vi "Consolidate Whitespace Text Lines.vi"(1 "Input":string) -> (0 "Output (consolidated whitespace lines)":string)   [LabVIEW 2023, in "Error Manager.lvlib"]
doc: "This VI replaces any set of two or more consecutive whitespace text lines with a single whitespace text line.\n\nIn this VI whitespace is defined as: spaces, tabs, carriage returns, and linefeeds.\n\n<B>Example 1</B>\nInput:\n\"\nHello World\n\n\nHello World\n\"\n\nOutput:\n\"\nHello World\n\nHello World\n\"\n\n<B>Example 2</B>\nInput:\n\"\nHello World\n\n\nHello World\n\n\n\n\nHello World\n\"\n\nOutput:\n\"\nHello World\n\nHello World\n\nHello World\n\""
uses:
  Error Manager.lvlib
  <vilib>/Utility/error.llb/whitespace.ctl
  <vilib>/Utility/error.llb/Trim Whitespace One-Sided.vi
  OpenG VIs/OpenG VIs.lvclass
panel:
  out "Whitespace Line Indexes":i32[](array[numeric])
  # "Development\nControls or indicators that are useful for development or testing, but which are not outputs of the VI."
  # "Input\nInputs to the VI"
  # "Output\nOutputs of the VI"
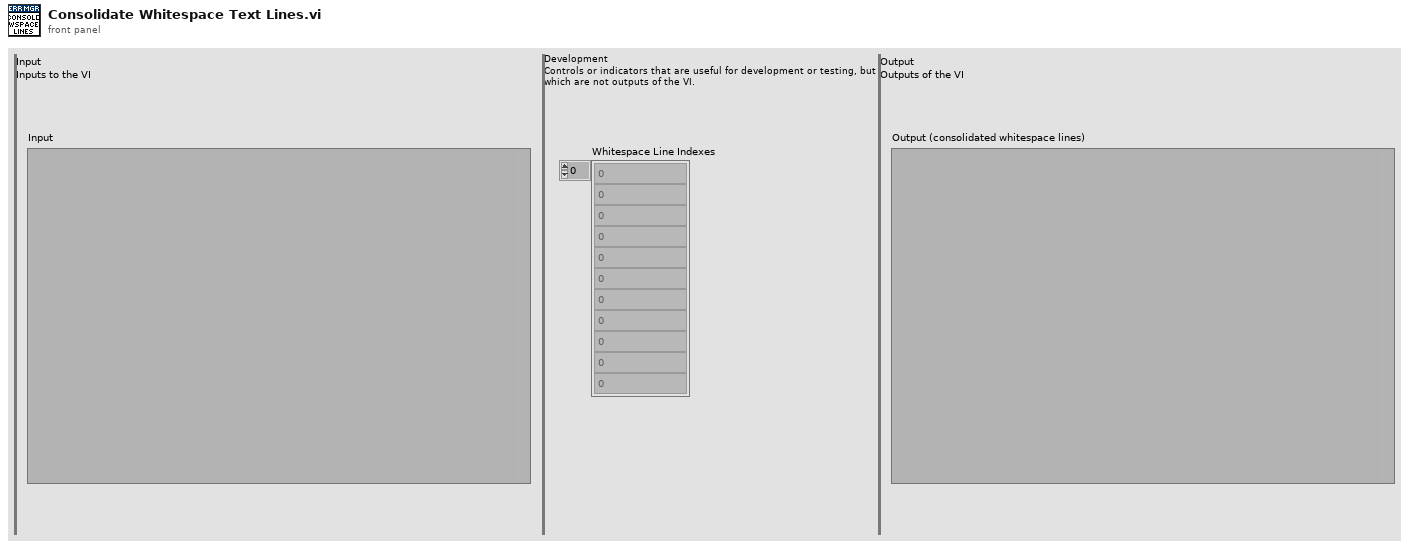
[diagram p1: front panel]
types:
  T1 = typedef "whitespace.ctl" = u16
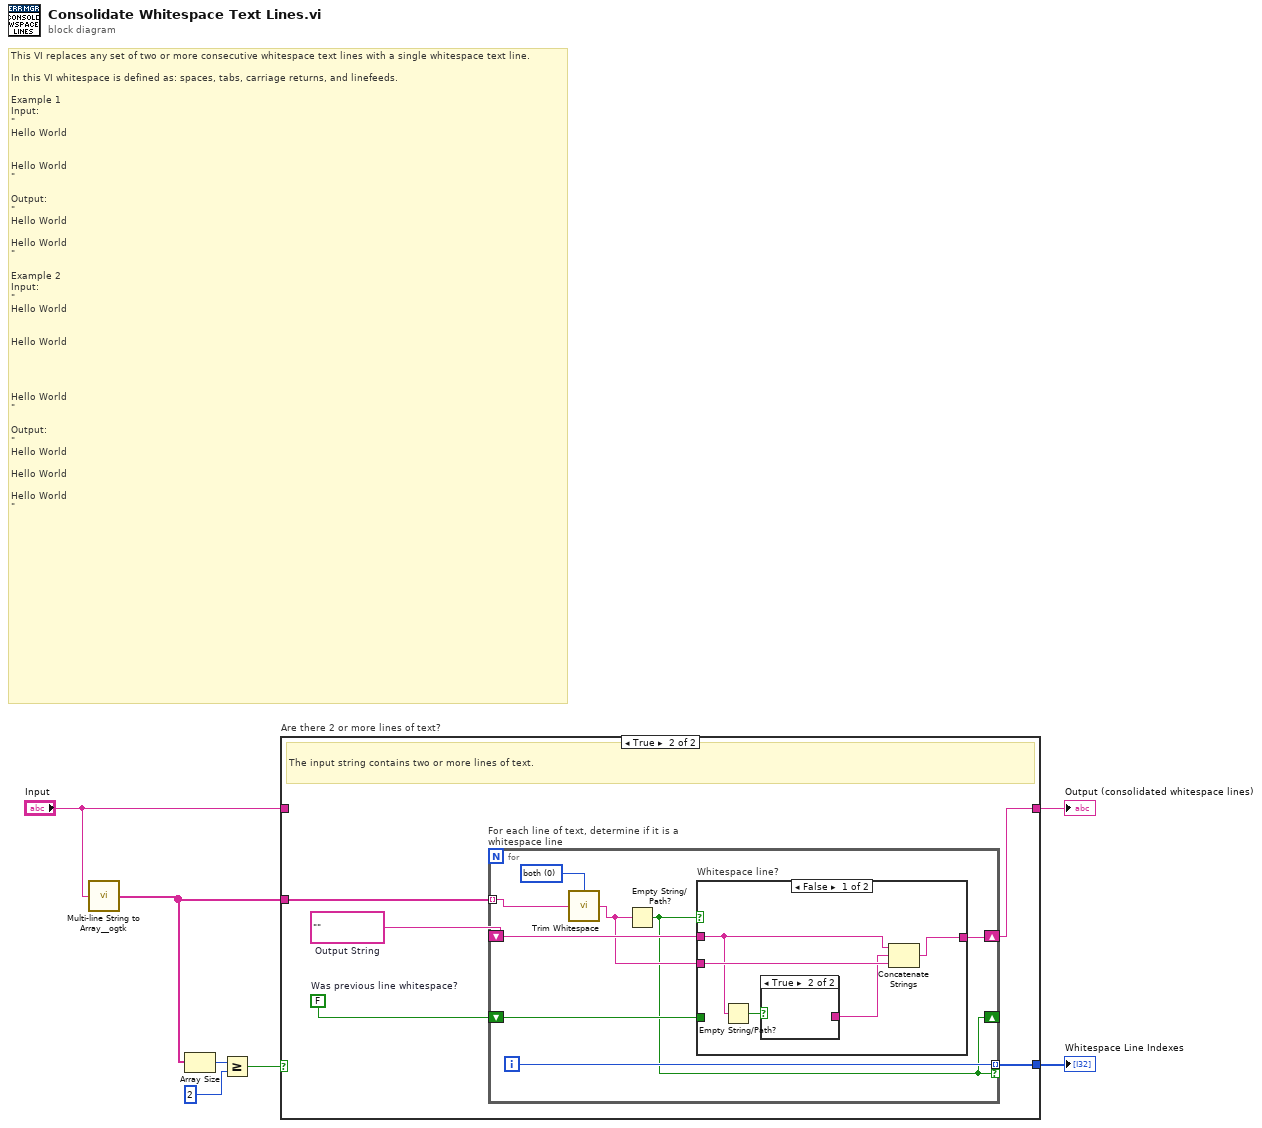
[diagram p0: block diagram]
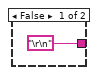
[diagram p3: hidden frame]
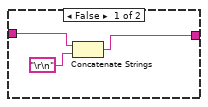
[diagram p5: hidden frame]
diagram:
  # "This VI replaces any set of two or more consecutive whitespace text lines with a single whitespace text line.\n\nIn this VI whitespace is defined as: spaces, tabs, carriage returns, and linefeeds.\n\nExample 1\nInput:\n\"\nHello World\n\n\nHello World\n\"\n\nOutput:\n\"\nHello World\n\nHello World\n\"\n\nExample 2\nInput:\n\"\nHello World\n\n\nHello World\n\n\n\n\nHello World\n\"\n\nOutput:\n\"\nHello World\n\nHello World\n\nHello World\n\""
  n1 = call "Multi-line String to Array__ogtk.vi"("string"="Input") -> ("lines"=w2:string[])
  n2 = Array Size(array=w2) -> (size(s)=w7:i32)
  n3 = Greater Or Equal?(x=w7, y=2) -> (x >= y?=w5:bool)
  n4 = case "Are there 2 or more lines of text?" shown="True" w5 {
    tunnel: "Input" -> [w8 _]
    tunnel: [w8 w9] -> w3
    tunnel: w2 -> [_ w13]
    tunnel: [_ w12] -> w1
    frame False {
      # "The input string is empty, or contains a single line of text. Pass it through unaltered."
    }
    frame True {
      w10 = FALSE  # Was previous line whitespace?
      w11 = ""  # Output String
      # "The input string contains two or more lines of text."
      n5 = for "For each line of text, determine if it is a whitespace line" {
        tunnel: w13 -> [w20] mode=indexing
        tunnel: [w19] -> w12 mode=indexing if=w14
        shift-right: [w16] -> w9
        shift-left: w11 -> [w18]
        shift-right: [w14] -> _
        shift-left: w10 -> [w15]
        i -> [w19]
        w21 = T1 0 items=["both", "start of string", "end of string"] ("location (both)")
        n6 = call <vilib>:"Trim Whitespace.vi"("string"=w20, "location (both)"=w21) -> ("trimmed string"=w17:string)
        n7 = Empty String/Path?(string/path=w17) -> (empty?=w14:bool)
        n8 = case "Whitespace line?" shown="False" w14 {
          tunnel: w18 -> [w23 w29]
          tunnel: w17 -> [w26 _]
          tunnel: [w25 w28] -> w16
          tunnel: w15 -> [_ w30]
          frame False {
            n9 = Empty String/Path?(string/path=w23) -> (empty?=w22:bool)
            n10 = case shown="True" w22 {
              tunnel: ["\r\n" _] -> w24
              frame False {
              }
              frame True {
              }
            }
            n11 = Concatenate Strings(w23, w24, w26) -> (w25:string)
          }
          frame True {
            n12 = case "Was previous line whitespace?" shown="True" w30 {
              tunnel: w29 -> [w33 w34]
              tunnel: [w31 w34] -> w28
              frame False {
                n13 = Concatenate Strings(w33, "\r\n") -> (w31:string)
              }
              frame True {
              }
            }
          }
        }
      }
    }
  }
  "Output (consolidated whitespace lines)" <- w3
  "Whitespace Line Indexes" <- w1
